vi "File_Setup.vi"(10 "File Name":string, 11 "Save Path":string) -> (3 "new file path (Not A Path if cancelled)":path)   [LabVIEW 2013]
uses:
  <vilib>/Utility/file.llb/Write To Spreadsheet File (string).vi
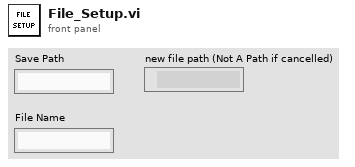
[diagram p1: front panel]
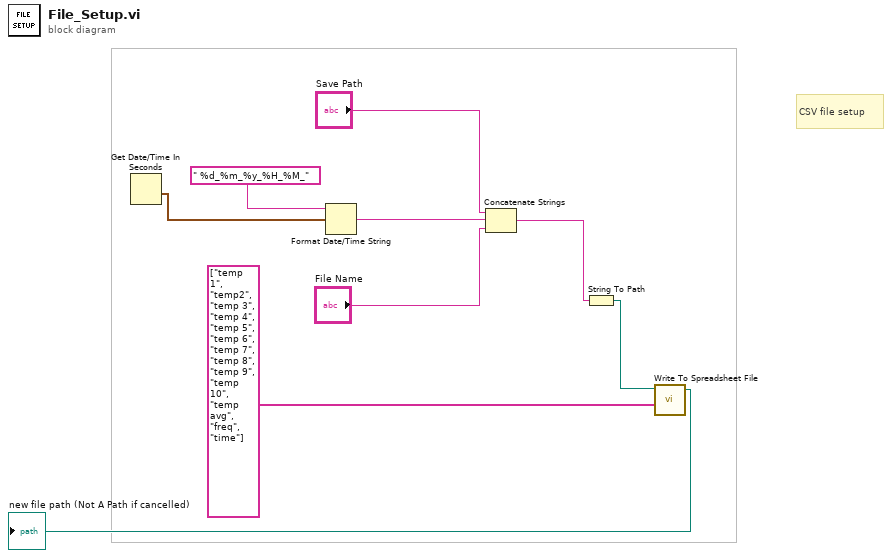
[diagram p0: block diagram]
diagram:
  # "CSV file setup"
  n1 = Get Date/Time In Seconds() -> (seconds since 1Jan1904=w2:timestamp)
  n2 = Format Date/Time String(time format string (%c)=" %d_%m_%y_%H_%M_", seconds (now)=w2) -> (date/time string=w4:string)  [unwired: 1 in]
  n3 = Concatenate Strings("Save Path", w4, "File Name") -> (w6:string)
  n4 = String To Path(string=w6) -> (path=w7:path)
  n5 = call-poly <vilib>:"Write To Spreadsheet File.vi"("1D data"=string[] ["temp 1", "temp2", "temp 3", "temp 4", "temp 5", "temp 6", "temp 7", "temp 8", "temp 9", "temp 10", "temp avg", "freq", "time"], "file path (dialog if empty)"=w7) -> ("new file path (Not A Path if cancelled)"=→"new file path (Not A Path if cancelled)":path)  [unwired: 6 in]
